vi "niRFUtil MEAS Compute IQ Imbalance.vi"(1 "Reference Signal In":T1 {"y" format="%.2f"; "dx" format="%^.2e"; "x0" format="%^.2e"}, 2 "Signal In":T1 {"y" format="%.2f"; "dx" format="%^.2e"; "x0" format="%^.2e"}) -> (0 "IQ Imbalance, dB":sgl format="%.2f")   [LabVIEW 2015, in "niRFUtil.lvlib"]
doc: "(c) Copyright 2006, National Instruments, Inc. This VI may not be duplicated, sold, or distributed without written consent from National Instruments."
uses:
  niRFUtil.lvlib
  Includes/niRFUtil INC Complex Waveform.ctl
  Includes/niRFUtil INC Complex Array.ctl
  <vilib>/Analysis/5stat.llb/RMS (DBL).vi
  <vilib>/Analysis/NI_AALPro.lvlib
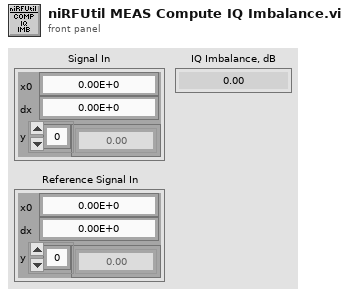
[diagram p1: front panel]
types:
  T1 = typedef "niRFUtil.lvlib/niRFUtil INC Complex Waveform.ctl" = cluster{"x0":dbl, "dx":dbl, "y":T2}
  T2 = typedef "niRFUtil.lvlib/niRFUtil INC Complex Array.ctl" = csg[]
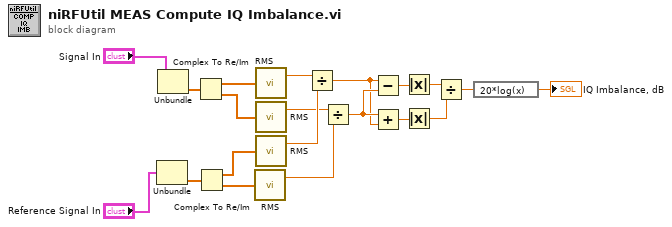
[diagram p0: block diagram]
diagram:
  n1 = Unbundle("Reference Signal In") -> ("y"=w17:T2)  [unwired: 2 out]
  n2 = Unbundle("Signal In") -> ("y"=w18:T2)  [unwired: 2 out]
  n3 = Complex To Re/Im(x + iy=w18) -> (x=w16:sgl[], y=w15:sgl[])
  n4 = Complex To Re/Im(x + iy=w17) -> (x=w14:sgl[], y=w13:sgl[])
  n5 = call-poly <vilib>:"RMS.vi"("X"=w13) -> ("rms value"=w9:dbl)  [unwired: 1 out]
  n6 = call-poly <vilib>:"RMS.vi"("X"=w16) -> ("rms value"=w12:dbl)  [unwired: 1 out]
  n7 = call-poly <vilib>:"RMS.vi"("X"=w15) -> ("rms value"=w10:dbl)  [unwired: 1 out]
  n8 = call-poly <vilib>:"RMS.vi"("X"=w14) -> ("rms value"=w11:dbl)  [unwired: 1 out]
  n9 = Divide(x=w12, y=w11) -> (x/y=w7:dbl)
  n10 = Divide(x=w10, y=w9) -> (x/y=w8:dbl)
  n11 = Subtract(x=w7, y=w8) -> (x-y=w6:dbl)
  n12 = Add(x=w8, y=w7) -> (x+y=w5:dbl)
  n13 = Absolute Value(x=w6) -> (abs(x)=w4:dbl)
  n14 = Absolute Value(x=w5) -> (abs(x)=w3:dbl)
  n15 = Divide(x=w4, y=w3) -> (x/y=w2:dbl)
  n16 = expression code="20*log(x)"(w2) -> (→"IQ Imbalance, dB":dbl)
